vi "Setup Environment.vi"(6 "working directory":path=path "", 8 "error in (no error)":errorcluster, 11 "PythonPlotter in":refnum<class "PythonPlotter.lvclass">) -> (0 "error out":errorcluster, 3 "PythonPlotter out":refnum<class "PythonPlotter.lvclass">)   [LabVIEW 2024, in "PythonPlotter.lvclass"]
uses:
  PythonPlotter.lvclass
  PythonPlotter.lvclass/PythonPlotter.ctl
panel:
  out "return code":i32
  out "standard error":string
  out "standard output":string
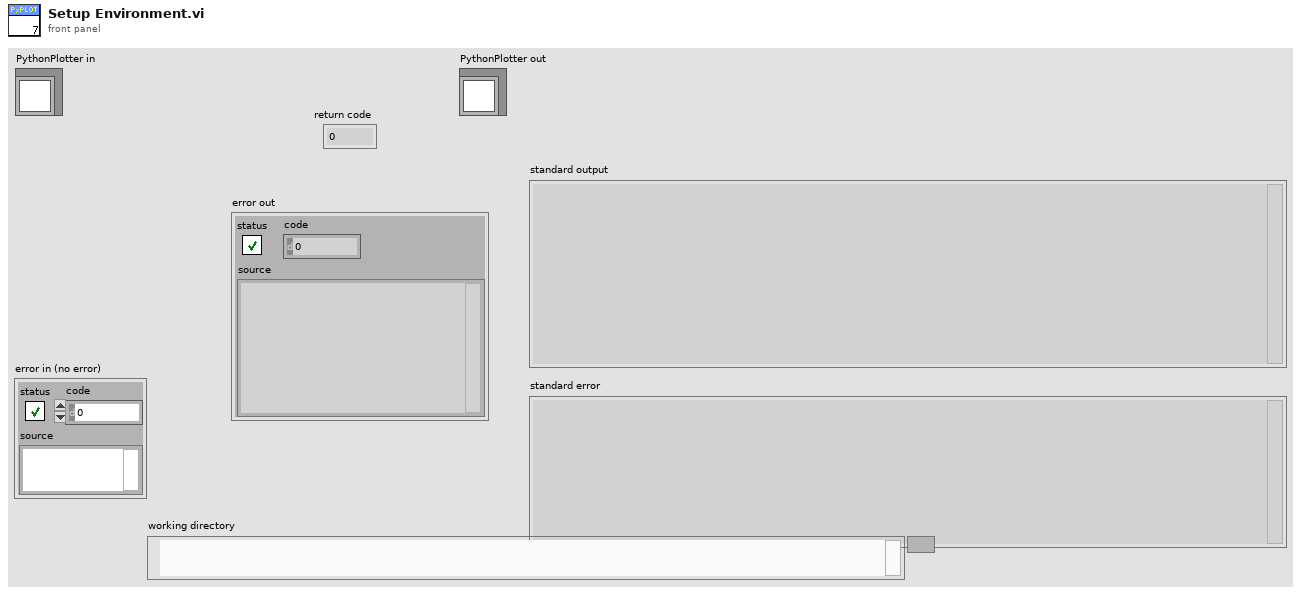
[diagram p1: front panel]
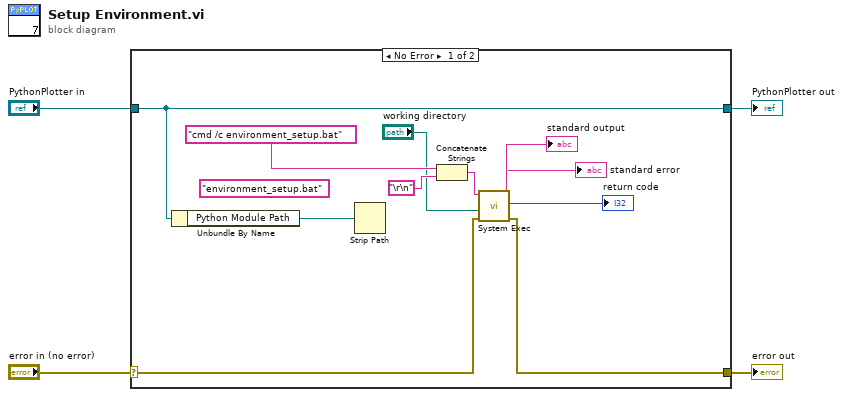
[diagram p0: block diagram]
diagram:
  n1 = case shown="No Error" "error in (no error)" {
    selector: "error in (no error)" -> [w10 w17]
    tunnel: [w9 w17] -> w3
    tunnel: [w15 w16] -> w1
    tunnel: "PythonPlotter in" -> [w15 w16]
    frame No Error {
      (unwired) "environment_setup.bat" ("command line")
      n2 = Unbundle By Name(w15) -> ("Python Module Path"=w14:path)
      n3 = Strip Path(path=w14) -> ()  [unwired: 2 out]
      n4 = Concatenate Strings("cmd /c environment_setup.bat" ("command line"), "\r\n") -> (w6:string)
      n5 = call <vilib>:"System Exec.vi"("error in (no error)"=w10, "working directory"="working directory", "command line"=w6) -> ("error out"=w9:errorcluster, "return code"=→"return code":i32, "standard error"=→"standard error":string, "standard output"=→"standard output":string)  [unwired: 5 in]
    }
    frame Error {
    }
  }
  "error out" <- w3
  "PythonPlotter out" <- w1
